vi "c Spark Get Periodic Status6.vi"(8 "error in (no error)":errorcluster, 10 "rawframe":T1, 11 "handle":T2) -> (0 "error out":errorcluster, 1 "function return":T3, 2 "rawframe out":T1, 3 "handle out":T2)   [LabVIEW 2023, in "REVLibDriver.lvlib"]
doc: "c_REVLib_ErrorCode c_Spark_GetPeriodicStatus6(\n c_Spark_handle handle, c_Spark_PeriodicStatus6* rawframe);"
uses:
  REVLibDriver.lvlib
  REVLibDriver.dll
  <vilib>/Custom Controls/c_Spark_handle.ctl
  subvi/RevLibError.ctl
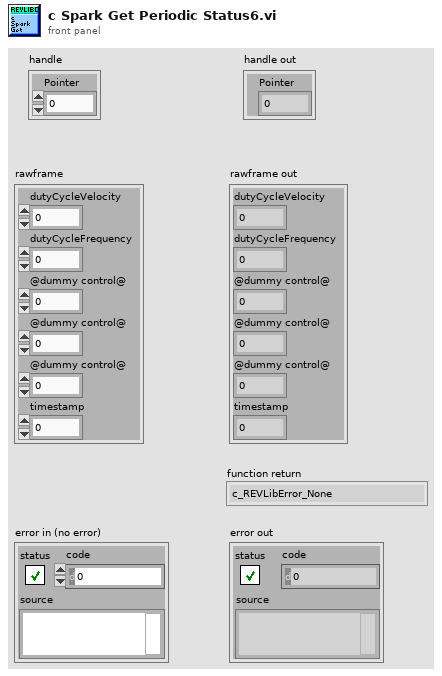
[diagram p1: front panel]
types:
  T1 = cluster{"dutyCycleVelocity":sgl, "dutyCycleFrequency":u8, "@dummy control@":i8, "@dummy control@":i8, "@dummy control@":i8, "timestamp":u64}
  T2 = typedef "REVLibDriver.lvlib/c_Spark_handle.ctl" = cluster{"Pointer":u32}
  T3 = typedef "REVLibDriver.lvlib/RevLibError.ctl" = enum16{"c_REVLibError_None", "c_REVLibError_General", "c_REVLibError_CANTimeout", "c_REVLibError_NotImplemented", "c_REVLibError_HAL", "c_REVLibError_CantFindFirmware", "c_REVLibError_FirmwareTooOld", "c_REVLibError_FirmwareTooNew", "c_REVLibError_ParamInvalidID", "c_REVLibError_ParamMismatchType", "c_REVLibError_ParamAccessMode", "c_REVLibError_ParamInvalid", "c_REVLibError_ParamNotImplementedDeprecated", "c_REVLibError_FollowConfigMismatch", "c_REVLibError_Invalid", "c_REVLibError_SetpointOutOfRange", "c_REVLibError_Unknown", "c_REVLibError_CANDisconnected", "c_REVLibError_DuplicateCANId", "c_REVLibError_InvalidCANId", "c_REVLibError_SparkMaxDataPortAlreadyConfiguredDifferently", "c_REVLibError_SparkFlexBrushedWithoutDock", "c_REVLibError_NumCodes"}
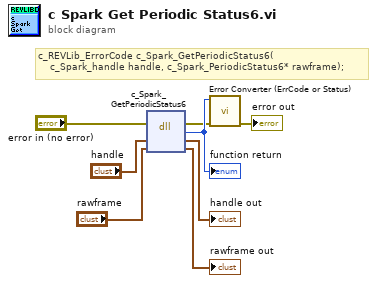
[diagram p0: block diagram]
diagram:
  # "c_REVLib_ErrorCode c_Spark_GetPeriodicStatus6(\n    c_Spark_handle handle, c_Spark_PeriodicStatus6* rawframe);"
  n1 = dll-call lib="REVLibDriver.*" fn="c_Spark_GetPeriodicStatus6"(error in="error in (no error)", "handle"="handle", "rawframe"="rawframe") -> (error out=w2:errorcluster, w8:u32, "handle"=→"handle out":T2, "rawframe"=→"rawframe out":T1)  [unwired: 2 in, 1 out]
  "function return" <- w8
  n2 = call "Error Converter (ErrCode or Status).vi"("error in (no error)"=w2, "error code"=w8) -> ("error out"=→"error out":errorcluster)  [unwired: 9 in]
